vi "test Timeout Is Total - Not Per Item (Call and Collect).vi"(8 "error in (no error)":errorcluster, 11 "TestCase in":refnum<class "Wait On All Future Tests.lvclass">) -> (0 "error out":errorcluster, 3 "TestCase out":refnum<class "Wait On All Future Tests.lvclass">)   [LabVIEW 2017, in "Wait On All Future Tests.lvclass"]
uses:
  Wait On All Future Tests.lvclass
  <vilib>/addons/_JKI Toolkits/VI Tester/TestCase.llb/TestCase.lvclass
  Futures/Futures.lvlib
  Futures/Future/Future.lvclass
  Futures/Promise/Promise.lvclass
  C:/Program Files (x86)/National Instruments/LabVIEW 2017/vi.lib/addons/_JKI Toolkits/VI Tester/TestCase.llb/TestCase.lvclass
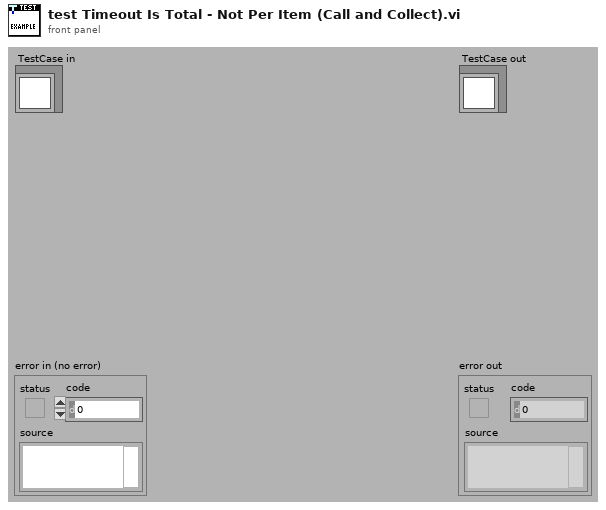
[diagram p1: front panel]
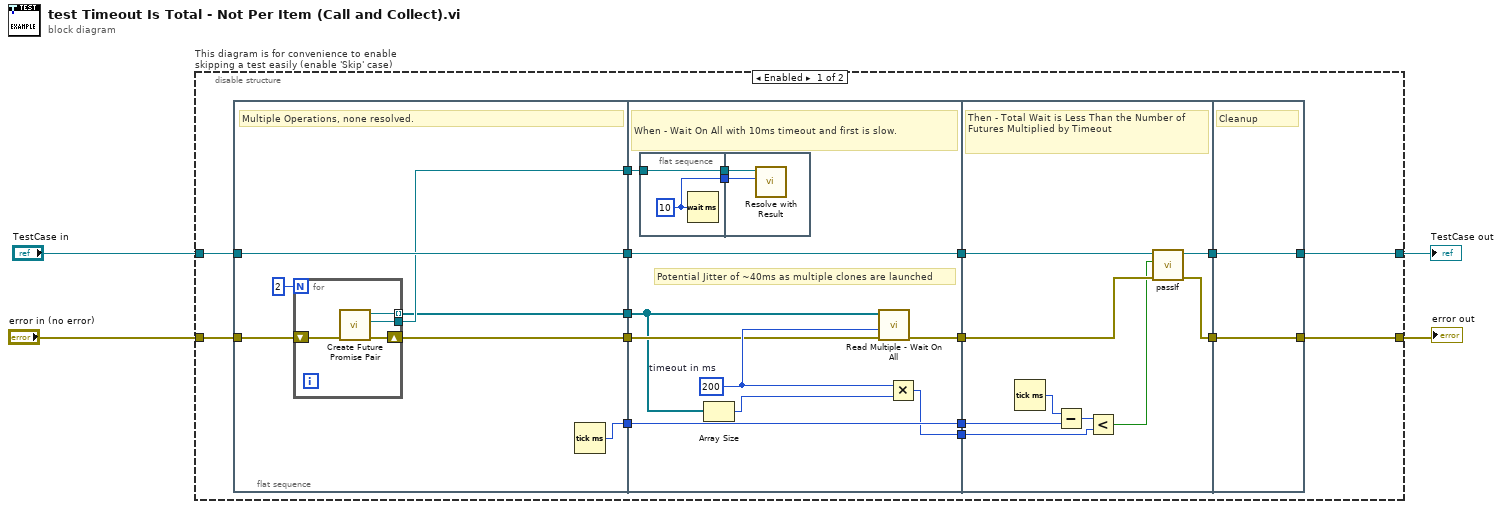
[diagram p0: block diagram]
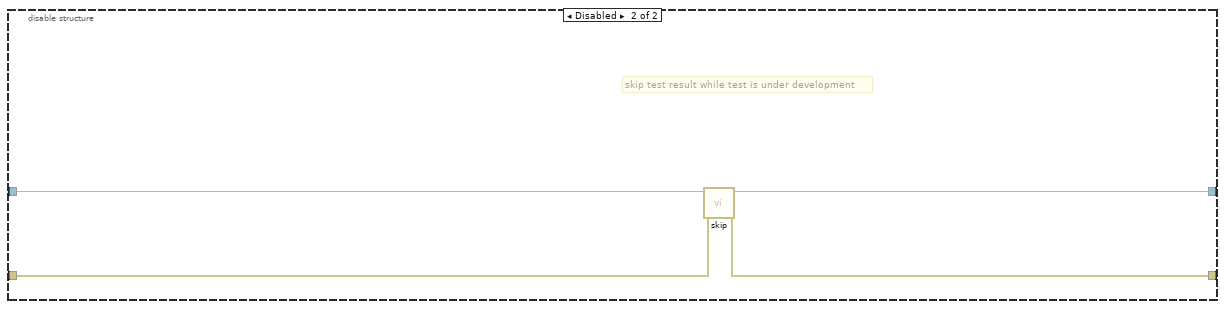
[diagram p2: hidden frame]
diagram:
  n1 = disable-structure "This diagram is for convenience to enable skipping a test easily (enable 'Skip' case)" shown="Enabled" {
    disable-tunnel: "TestCase in" -> [w15 w60]
    disable-tunnel: [w13 w58] -> w1
    disable-tunnel: [w12 w59] -> w3
    disable-tunnel: "error in (no error)" -> [w14 w57]
    frame Enabled {
      n2 = flat-sequence {
        tunnel: w14 -> [w25]
        tunnel: w15 -> [w26]
        tunnel: [w26] -> w19
        tunnel: [w24] -> w10
        tunnel: [w23] -> w8
        tunnel: [w21] -> w6
        tunnel: [w20] -> w5
        tunnel: [w41] -> w18
        tunnel: w19 -> [w41]
        tunnel: [w40] -> w11
        tunnel: w10 -> [w39]
        tunnel: [w39] -> w9
        tunnel: w8 -> [w37]
        tunnel: [w33] -> w7
        tunnel: w6 -> [w31]
        tunnel: w5 -> [w32]
        tunnel: [w51] -> w17
        tunnel: [w49] -> w16
        tunnel: w18 -> [w52]
        tunnel: w11 -> [w50]
        tunnel: w9 -> [w53]
        tunnel: w7 -> [w46]
        tunnel: [w55] -> w12
        tunnel: [w56] -> w13
        tunnel: w17 -> [w56]
        tunnel: w16 -> [w55]
        frame #0 {
          # "Multiple Operations, none resolved."
          n3 = for {
            N: 2 -> [_]
            tunnel: [w29] -> w23
            tunnel: [w28] -> w21 mode=indexing
            shift-right: [w27] -> w20
            shift-left: w25 -> [w30]
            n4 = call "Create Future Promise Pair.vi"("error in (no error)"=w30) -> ("error out"=w27:errorcluster, "Promise out"=w29:refnum<class "Promise.lvclass">, "Future out"=w28:refnum<class "Future.lvclass">)  [unwired: 8 in]
          }
          n5 = Tick Count (ms)() -> (millisecond timer value=w24:u32)
        }
        frame #1 {
          w35 = 200  # timeout in ms
          # "Potential Jitter of ~40ms as multiple clones are launched"
          # "When - Wait On All with 10ms timeout and first is slow."
          n6 = flat-sequence {
            tunnel: [w43] -> w38
            tunnel: w37 -> [w42]
            tunnel: [w42] -> w36
            tunnel: w38 -> [w45]
            tunnel: w36 -> [w44]
            frame #0 {
              w43 = u32 10 ("milliseconds to wait")
              n7 = Wait (ms)(milliseconds to wait=w43) -> ()  [unwired: 1 out]
            }
            frame #1 {
              n8 = call "Resolve with Result.vi"("Result"=w45, "Promise in"=w44) -> ()  [unwired: 9 in, 1 out]
            }
          }
          n9 = Array Size(array=w31) -> (size(s)=w34:i32)
          n10 = call "Read Multiple - Wait On All.vi"("error in (no error)"=w32, "timeout in ms (60 sec)"=w35, "Futures in"=w31) -> ("error out"=w40:errorcluster)  [unwired: 5 in, 3 out]
          n11 = Multiply(x=w35, y=w34) -> (x*y=w33:i32)
        }
        frame #2 {
          # "Then - Total Wait is Less Than the Number of Futures Multiplied by Timeout"
          n12 = Tick Count (ms)() -> (millisecond timer value=w54:u32)
          n13 = Subtract(x=w54, y=w53) -> (x-y=w48:u32)
          n14 = Less?(x=w48, y=w46) -> (x < y?=w47:bool)
          n15 = call-dynamic "passIf.vi"("error in (no error)"=w50, "pass"=w47, "TestCase in"=w52) -> ("error out"=w49:errorcluster, "TestCase out"=w51:refnum<class "Wait On All Future Tests.lvclass">)  [unwired: 7 in]
        }
        frame #3 {
          # "Cleanup"
        }
      }
    }
    frame Disabled {
      # "skip test result while test is under development"
      n16 = call <vilib>:"skip.vi"("error in (no error)"=w57, "TestCase in"=w60) -> ("error out"=w59:errorcluster, "TestCase out"=w58:refnum<class "Wait On All Future Tests.lvclass">)  [unwired: 8 in]
    }
  }
  "error out" <- w3
  "TestCase out" <- w1
